vi "CheckLimitSwitches.vi"(8 "error in (no error)":errorcluster caption="Fehler (Eingang, kein Fehler)", 10 "BoolArrayIn":bool[](array[boolean]), 11 "NumberOfAxes":u8) -> (0 "error out":errorcluster, 3 "LimitsOutput":T1[](array[typedef]))   [LabVIEW 2018]
uses:
  Axis_Switch.ctl
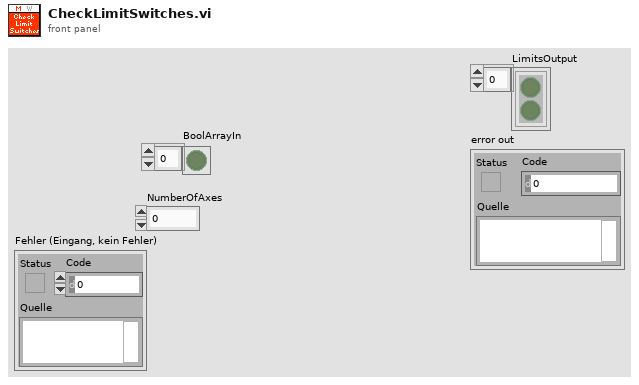
[diagram p1: front panel]
types:
  T1 = typedef "Axis_Switch.ctl" = cluster{"E0":bool, "EE":bool}
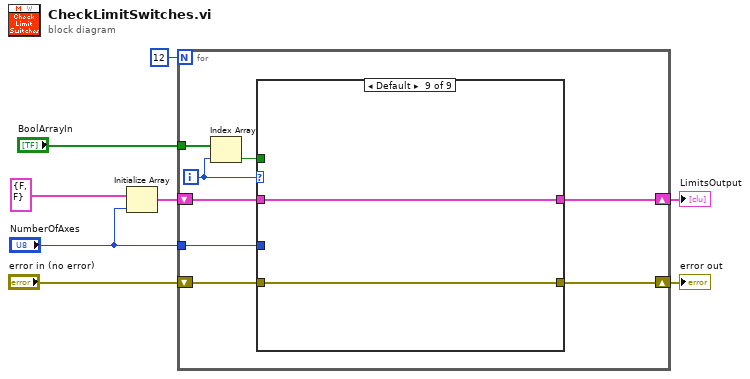
[diagram p0: block diagram]
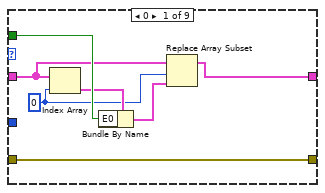
[diagram p2: hidden frame]
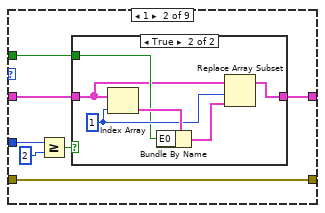
[diagram p3: hidden frame]
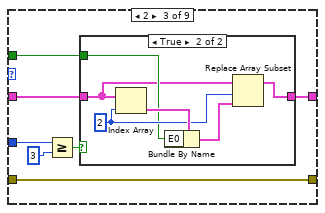
[diagram p5: hidden frame]
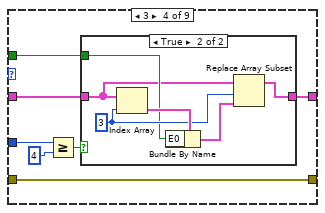
[diagram p7: hidden frame]
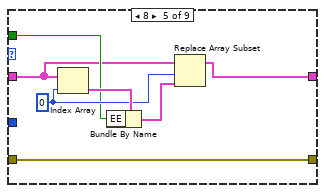
[diagram p9: hidden frame]
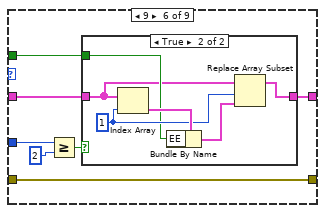
[diagram p10: hidden frame]
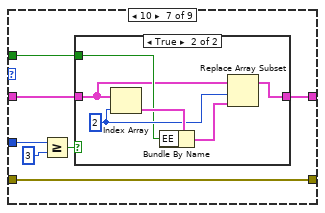
[diagram p12: hidden frame]
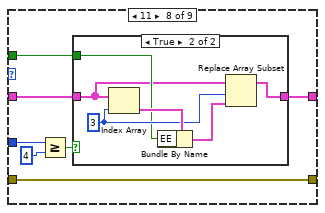
[diagram p14: hidden frame]
diagram:
  n1 = Initialize Array(T1 {"E0"=FALSE, "EE"=FALSE} ("Switch"), "NumberOfAxes") -> (w5:T1[])
  n2 = for {
    N: 12 -> [_]
    tunnel: "BoolArrayIn" -> [w16]
    shift-right: [w12] -> w4
    shift-left: w5 -> [w13]
    tunnel: "NumberOfAxes" -> [w11]
    shift-right: [w9] -> w1
    shift-left: "error in (no error)" -> [w10]
    i -> [w15]
    n3 = Index Array(array=w16, index=w15) -> (element=w14:bool)
    n4 = case shown="Default" w15 {
      tunnel: w14 -> [w23 w30 w42 w56 w69 w77 w91 w105 _]
      tunnel: w13 -> [w22 w29 w41 w55 w68 w76 w90 w104 w116]
      tunnel: [w21 w25 w39 w53 w67 w74 w88 w102 w116] -> w12
      tunnel: w11 -> [_ w27 w40 w54 _ w75 w89 w103 _]
      tunnel: [w17 w24 w38 w52 w66 w73 w87 w101 w115] -> w9
      tunnel: w10 -> [w17 w24 w38 w52 w66 w73 w87 w101 w115]
      frame 0 {
        w18 = 0 ("Index")
        n5 = Index Array(array=w22, index=w18) -> (element=w20:T1)
        n6 = Bundle By Name(cluster=w20, "E0"=w23) -> (w19:T1)
        n7 = Replace Array Subset(array=w22, new element=w19, index=w18) -> (w21:T1[])
      }
      frame 1 {
        n8 = Greater Or Equal?(x=w27, y=u8 2) -> (x >= y?=w28:bool)
        n9 = case shown="True" w28 {
          tunnel: w30 -> [_ w34]
          tunnel: w29 -> [w31 w33]
          tunnel: [w31 w32] -> w25
          frame False {
          }
          frame True {
            w35 = 1 ("Index")
            n10 = Index Array(array=w33, index=w35) -> (element=w37:T1)
            n11 = Bundle By Name(cluster=w37, "E0"=w34) -> (w36:T1)
            n12 = Replace Array Subset(array=w33, new element=w36, index=w35) -> (w32:T1[])
          }
        }
      }
      frame 2 {
        n13 = Greater Or Equal?(x=w40, y=u8 3) -> (x >= y?=w44:bool)
        n14 = case shown="True" w44 {
          tunnel: w42 -> [_ w48]
          tunnel: w41 -> [w45 w47]
          tunnel: [w45 w46] -> w39
          frame False {
          }
          frame True {
            w49 = 2 ("Index")
            n15 = Index Array(array=w47, index=w49) -> (element=w51:T1)
            n16 = Bundle By Name(cluster=w51, "E0"=w48) -> (w50:T1)
            n17 = Replace Array Subset(array=w47, new element=w50, index=w49) -> (w46:T1[])
          }
        }
      }
      frame 3 {
        n18 = Greater Or Equal?(x=w54, y=u8 4) -> (x >= y?=w58:bool)
        n19 = case shown="True" w58 {
          tunnel: w56 -> [_ w62]
          tunnel: w55 -> [w59 w61]
          tunnel: [w59 w60] -> w53
          frame False {
          }
          frame True {
            w63 = 3 ("Index")
            n20 = Index Array(array=w61, index=w63) -> (element=w65:T1)
            n21 = Bundle By Name(cluster=w65, "E0"=w62) -> (w64:T1)
            n22 = Replace Array Subset(array=w61, new element=w64, index=w63) -> (w60:T1[])
          }
        }
      }
      frame 8 {
        w70 = 0 ("Index")
        n23 = Index Array(array=w68, index=w70) -> (element=w72:T1)
        n24 = Bundle By Name(cluster=w72, "EE"=w69) -> (w71:T1)
        n25 = Replace Array Subset(array=w68, new element=w71, index=w70) -> (w67:T1[])
      }
      frame 9 {
        n26 = Greater Or Equal?(x=w75, y=u8 2) -> (x >= y?=w79:bool)
        n27 = case shown="True" w79 {
          tunnel: w77 -> [_ w83]
          tunnel: w76 -> [w80 w82]
          tunnel: [w80 w81] -> w74
          frame False {
          }
          frame True {
            w84 = 1 ("Index")
            n28 = Index Array(array=w82, index=w84) -> (element=w86:T1)
            n29 = Bundle By Name(cluster=w86, "EE"=w83) -> (w85:T1)
            n30 = Replace Array Subset(array=w82, new element=w85, index=w84) -> (w81:T1[])
          }
        }
      }
      frame 10 {
        n31 = Greater Or Equal?(x=w89, y=u8 3) -> (x >= y?=w93:bool)
        n32 = case shown="True" w93 {
          tunnel: w91 -> [_ w97]
          tunnel: w90 -> [w94 w96]
          tunnel: [w94 w95] -> w88
          frame False {
          }
          frame True {
            w98 = 2 ("Index")
            n33 = Index Array(array=w96, index=w98) -> (element=w100:T1)
            n34 = Bundle By Name(cluster=w100, "EE"=w97) -> (w99:T1)
            n35 = Replace Array Subset(array=w96, new element=w99, index=w98) -> (w95:T1[])
          }
        }
      }
      frame 11 {
        n36 = Greater Or Equal?(x=w103, y=u8 4) -> (x >= y?=w107:bool)
        n37 = case shown="True" w107 {
          tunnel: w105 -> [_ w111]
          tunnel: w104 -> [w108 w110]
          tunnel: [w108 w109] -> w102
          frame False {
          }
          frame True {
            w112 = 3 ("Index")
            n38 = Index Array(array=w110, index=w112) -> (element=w114:T1)
            n39 = Bundle By Name(cluster=w114, "EE"=w111) -> (w113:T1)
            n40 = Replace Array Subset(array=w110, new element=w113, index=w112) -> (w109:T1[])
          }
        }
      }
      frame Default {
      }
    }
  }
  "LimitsOutput" <- w4
  "error out" <- w1
